vi "MainConfigUI.vi"(8 "ConfigWindowName":string="Config", 9 "Communication Data":T2, 10 "Notifiers":T3, 11 "BaseDashPath":path) -> ()   [LabVIEW 2015]
uses:
  General/RemoteFiles/connectionData.ctl
  ConfigXML/typedefs/MotorControl.ctl
  ConfigXML/typedefs/EncoderControl.ctl
  ConfigXML/typedefs/PIDControl.ctl
  ConfigXML/typedefs/SetpointArrControl.ctl
  ConfigXML/src/ConfigXMLControl.ctl
panel:
  out "Config Currently on Target":string
  out "windowName":string
  in  "ViewCfgOnBot":bool
  in  "ULConfigtoRIO":bool
  in  "LoadConfig":bool
  in  "SaveConfig":bool
  in  "Tab Control":enum32{"IntakeLift", "ChooChoo"}(tab)
  in  "IntakeLift":T8
  in  "ChooChoo":T8
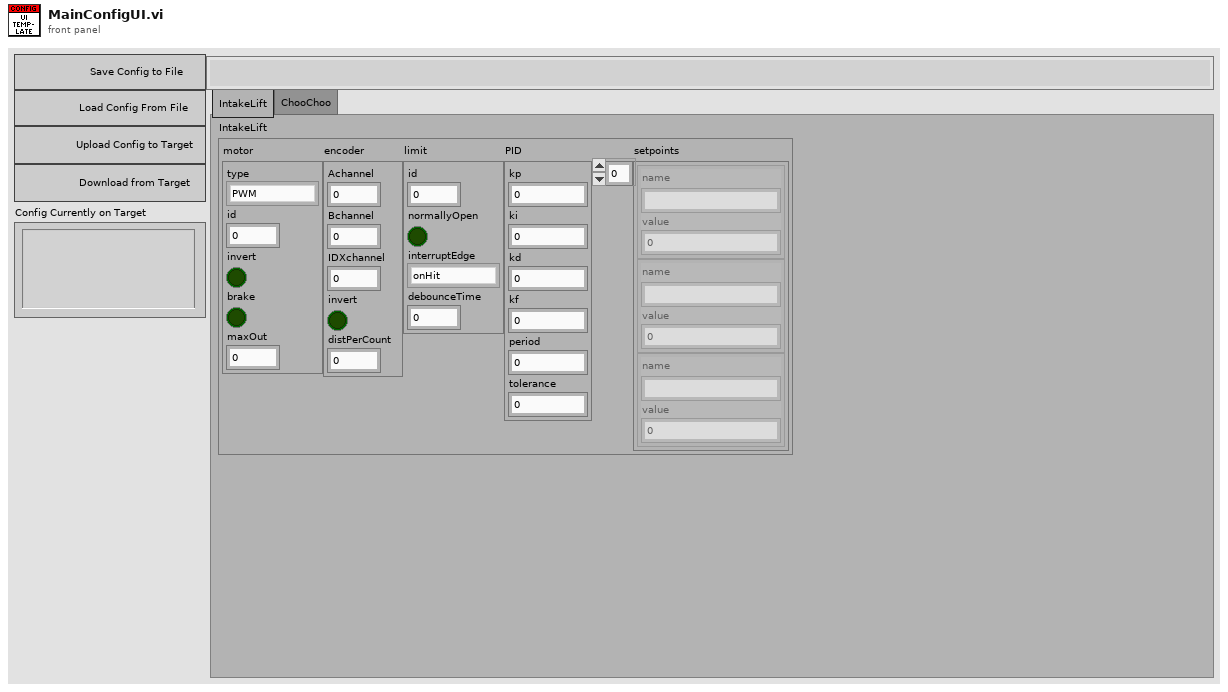
[diagram p1: front panel]
types:
  T1 = typedef "connectionData.ctl" = cluster{"host":string, "user":string, "password":string, "port":u16}
  T2 = cluster{"TargetFilePath":string, "ConnectionData":T1}
  T3 = cluster{"IP_Notifier":refnum<notifier>, "WindowNotifier":refnum<notifier>, "Stop_Notifier":refnum<notifier>}
  T4 = typedef "MotorControl.ctl" = cluster{"type":enum16{"PWM", "CANTalon"}, "id":i32, "invert":bool, "brake":bool, "maxOut":dbl}
  T5 = typedef "EncoderControl.ctl" = cluster{"Achannel":i32, "Bchannel":i32, "IDXchannel":i32, "invert":bool, "distPerCount":dbl}
  T6 = typedef "PIDControl.ctl" = cluster{"kp":dbl, "ki":dbl, "kd":dbl, "kf":dbl, "period":dbl, "tolerance":dbl}
  T7 = typedef "SetpointArrControl.ctl" = cluster{"name":string, "value":dbl}[]
  T8 = cluster{"motor":T4, "encoder":T5, "limit":cluster{"id":i32, "normallyOpen":bool, "interruptEdge":enum16{"onHit", "onRelease", "both"}, "debounceTime":dbl}, "PID":T6, "setpoints":T7}
  T9 = typedef "ConfigXMLControl.ctl" = cluster{"ViewCfgOnTarget":refnum<vi>, "ULConfigtoTarget":refnum<vi>, "TabControl":refnum<vi>, "ConfigOnTarget":refnum<vi>, "LoadConfig":refnum<vi>, "SaveConfig":refnum<vi>, "Stop_Notifier":refnum<notifier>, "IP_Notifier":refnum<notifier>, "WindowNotifier":refnum<notifier>, "BaseDirectory":path, "TargetFilePath":string}
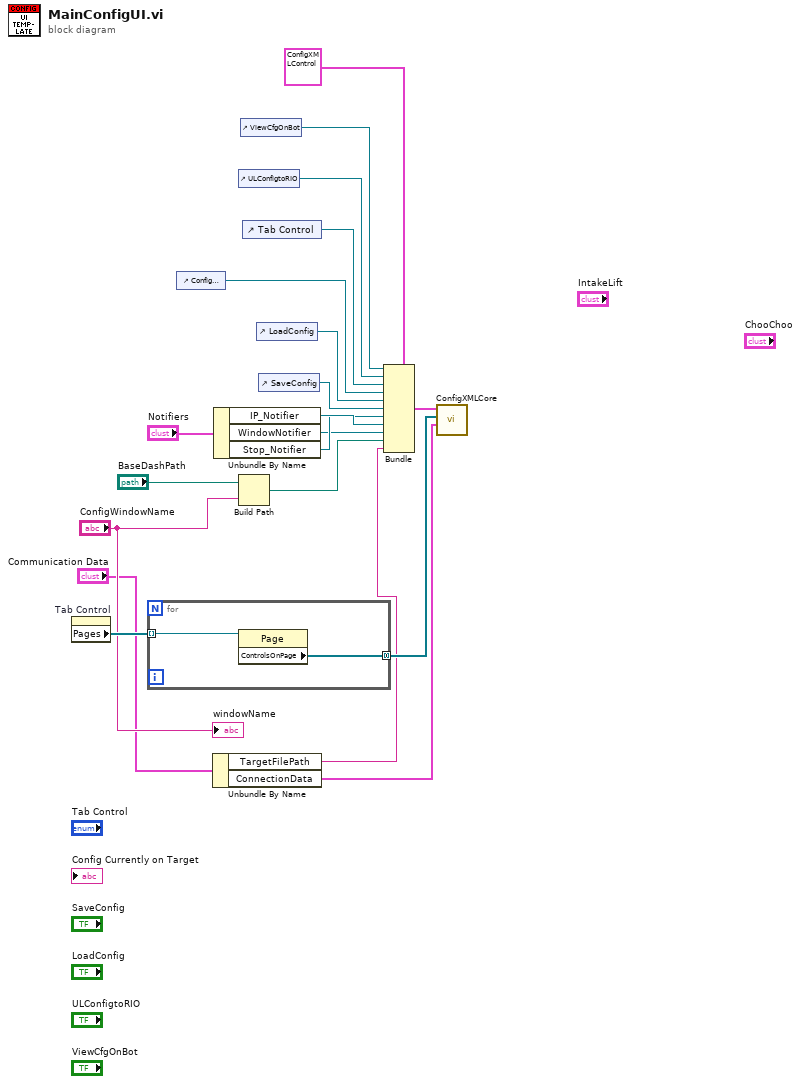
[diagram p0: block diagram]
diagram:
  n1 = property on="Tab Control" class="TabCtl (strict)"() -> ("Pages"=w20:refnum<vi>[])  [unwired: 2 in, 2 out]
  n2 = for {
    tunnel: w20 -> [w22] mode=indexing
    tunnel: [w21] -> w11 mode=concatenating
    n3 = property class="Page"(reference=w22) -> ("ControlsOnPage"=w21:refnum<vi>[])  [unwired: 1 in, 2 out]
  }
  n4 = control-ref of="Config Currently on Target"() -> (w9:refnum<vi>)
  n5 = Unbundle By Name("Communication Data") -> ("TargetFilePath"=w2:string, "ConnectionData"=w1:T1)
  n6 = Unbundle By Name("Notifiers") -> ("IP_Notifier"=w6:refnum<notifier>, "WindowNotifier"=w4:refnum<notifier>, "Stop_Notifier"=w5:refnum<notifier>)
  n7 = control-ref of="ULConfigtoRIO"() -> (w18:refnum<vi>)
  n8 = Build Path(base path="BaseDashPath", name or relative path="ConfigWindowName") -> (appended path=w14:path)
  n9 = control-ref of="ViewCfgOnBot"() -> (w19:refnum<vi>)
  n10 = control-ref of="Tab Control"() -> (w8:refnum<vi>)
  n11 = control-ref of="LoadConfig"() -> (w17:refnum<vi>)
  n12 = control-ref of="SaveConfig"() -> (w16:refnum<vi>)
  n13 = Bundle(cluster=T9 {"ViewCfgOnTarget"=refnum, "ULConfigtoTarget"=refnum, "TabControl"=refnum, "ConfigOnTarget"=refnum, "LoadConfig"=refnum, "SaveConfig"=refnum, "Stop_Notifier"=refnum, "IP_Notifier"=refnum, "WindowNotifier"=refnum, "BaseDirectory"=path "", "TargetFilePath"=""} ("output cluster"), "ViewCfgOnTarget"=w19, "ULConfigtoTarget"=w18, "TabControl"=w8, "ConfigOnTarget"=w9, "LoadConfig"=w17, "SaveConfig"=w16, "Stop_Notifier"=w5, "IP_Notifier"=w6, "WindowNotifier"=w4, "BaseDirectory"=w14, "TargetFilePath"=w2) -> (w12:T9)
  n14 = call "ConfigXMLCore.vi"("ConnectionData"=w1, "controlsToSave"=w11, "ConfigXMLControl"=w12) -> ()  [unwired: 9 in]
  "windowName" <- "ConfigWindowName"
